vi "ROVinput 30k subvi.vi"(0 "String":string) -> (1 "depth":dbl=-10.0 format="%.1f", 2 "altitude":dbl=999.0 format="%.1f", 3 "heading":dbl=700.0 format="%#.1f", 4 "yaw rate":dbl=100000.0 format="%#.1f")   [LabVIEW 2014]
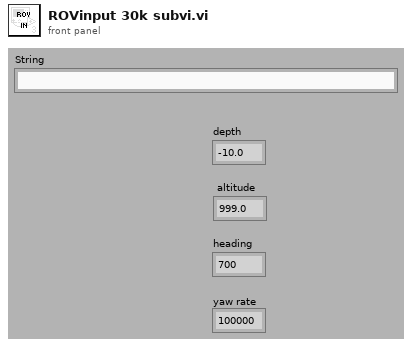
[diagram p1: front panel]
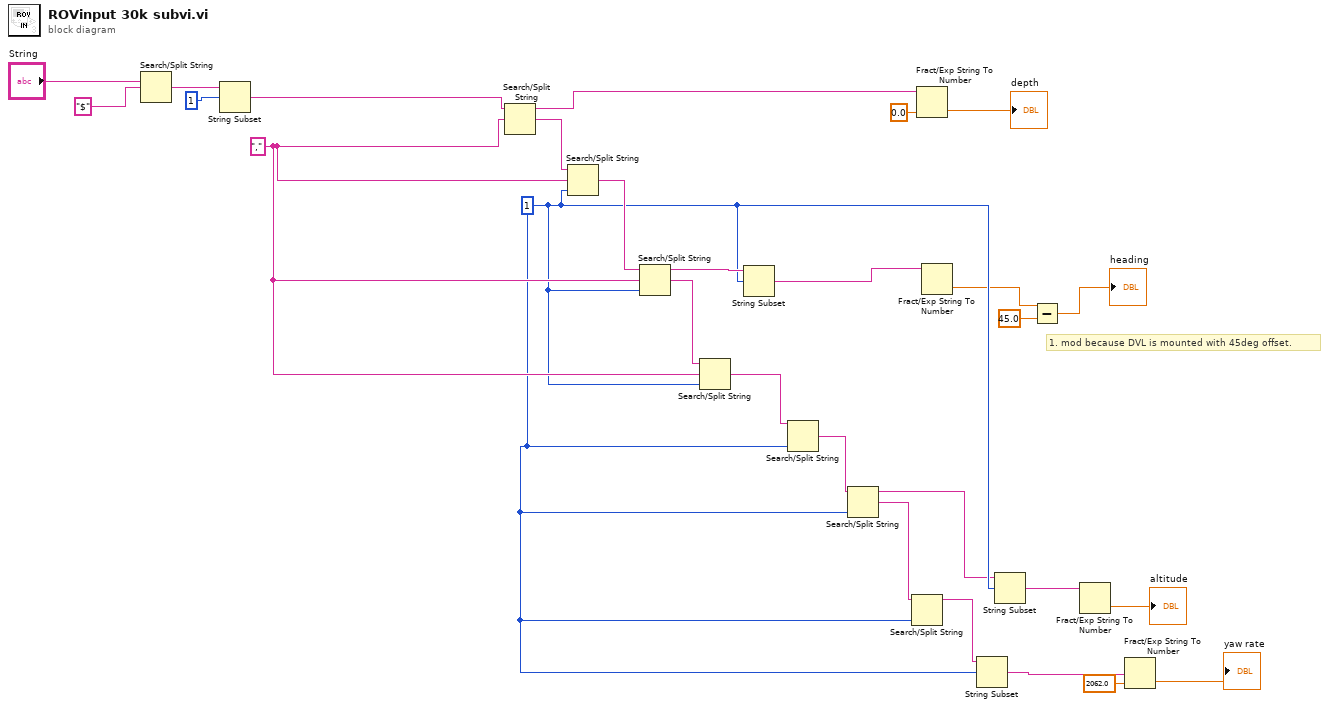
[diagram p0: block diagram]
diagram:
  w6 = 1
  w15 = ","
  # "1. mod because DVL is mounted with 45deg offset."
  n1 = Search/Split String(string="String", search string/char (-)="$") -> (match + rest of string=w18:string)  [unwired: 1 in, 2 out]
  n2 = String Subset(string=w18, offset (0)=1) -> (substring=w14:string)  [unwired: 1 in]
  n3 = Search/Split String(string=w14, search string/char (-)=w15) -> (substring before match=w23:string, match + rest of string=w20:string)  [unwired: 1 in, 1 out]
  n4 = Search/Split String(string=w20, search string/char (-)=w15, offset (0)=w6) -> (match + rest of string=w21:string)  [unwired: 2 out]
  n5 = Search/Split String(string=w21, search string/char (-)=w15, offset (0)=w6) -> (substring before match=w11:string, match + rest of string=w22:string)  [unwired: 1 out]
  n6 = Search/Split String(string=w22, search string/char (-)=w15, offset (0)=w6) -> (match + rest of string=w10:string)  [unwired: 2 out]
  n7 = String Subset(string=w11, offset (0)=w6) -> (substring=w25:string)  [unwired: 1 in]
  n8 = Search/Split String(string=w10, offset (0)=w6) -> (match + rest of string=w9:string)  [unwired: 1 in, 2 out]
  n9 = Search/Split String(string=w9, offset (0)=w6) -> (substring before match=w5:string, match + rest of string=w8:string)  [unwired: 1 in, 1 out]
  n10 = Search/Split String(string=w8, offset (0)=w6) -> (substring before match=w7:string)  [unwired: 1 in, 2 out]
  n11 = Fract/Exp String To Number(string=w23, default (0 dbl)=0.0 ("default (0 DBL)")) -> (number=→"depth":dbl)  [unwired: 2 in, 1 out]
  n12 = Fract/Exp String To Number(string=w25) -> (number=w2:dbl)  [unwired: 3 in, 1 out]
  n13 = String Subset(string=w7, offset (0)=w6) -> (substring=w27:string)  [unwired: 1 in]
  n14 = String Subset(string=w5, offset (0)=w6) -> (substring=w26:string)  [unwired: 1 in]
  n15 = Subtract(x=w2, y=45.0) -> (x-y=→"heading":dbl)
  n16 = Fract/Exp String To Number(string=w26) -> (number=→"altitude":dbl)  [unwired: 3 in, 1 out]
  n17 = Fract/Exp String To Number(string=w27, default (0 dbl)=2062.0 ("default (0 DBL)")) -> (number=→"yaw rate":dbl)  [unwired: 2 in, 1 out]
